vi "addEnumLiteral.vi"(8 "error in (no error)":errorcluster, 9 "enumerationLiteral":string, 10 "enumName":string, 11 "Enumeration in":refnum<class "Enumeration.lvclass">) -> (0 "error out":errorcluster, 3 "Enumeration out":refnum<class "Enumeration.lvclass">)   [LabVIEW 2016, in "Enumeration.lvclass"]
uses:
  Enumeration.lvclass
  Enumeration.lvclass/Enumeration.ctl
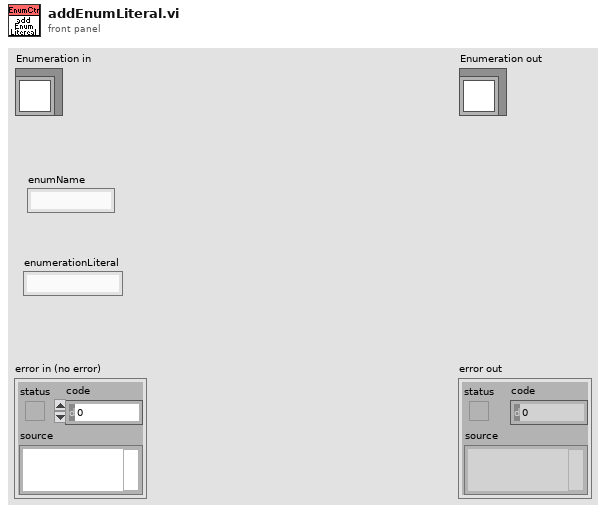
[diagram p1: front panel]
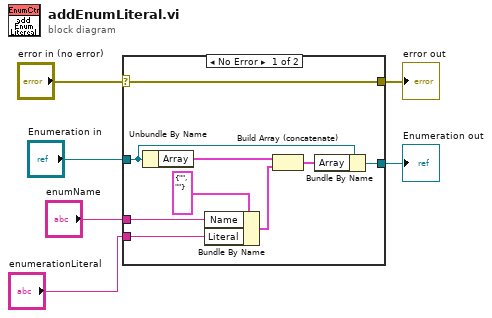
[diagram p0: block diagram]
diagram:
  n1 = case shown="No Error" "error in (no error)" {
    selector: "error in (no error)" -> [w15 w17]
    tunnel: [w15 w17] -> w5
    tunnel: [w11 w16] -> w3
    tunnel: "Enumeration in" -> [w10 w16]
    tunnel: "enumName" -> [w13 _]
    tunnel: "enumerationLiteral" -> [w12 _]
    frame No Error {
      n2 = Unbundle By Name(w10) -> ("Array"=w8:cluster{"Name":string, "Literal":string}[])
      n3 = Bundle By Name(cluster=cluster{"Name":string, "Literal":string} {"Name"="", "Literal"=""} ("Cluster"), "Name"=w13, "Literal"=w12) -> (w7:cluster{"Name":string, "Literal":string})
      n4 = Build Array (concatenate)(w8, w7) -> (w9:cluster{"Name":string, "Literal":string}[])
      n5 = Bundle By Name(cluster=w10, "Array"=w9) -> (w11:refnum<class "Enumeration.lvclass">)
    }
    frame Error {
    }
  }
  "error out" <- w5
  "Enumeration out" <- w3
